vi "Read Name.vi"(8 "error in (no error)":errorcluster, 11 "EmbeddedSMO in":refnum<class "Embedded UI.lvclass">) -> (0 "error out":errorcluster, 2 "Name":string, 3 "EmbeddedSMO out":refnum<class "Embedded UI.lvclass">)   [LabVIEW 2019, in "Embedded UI.lvclass"]
uses:
  Embedded UI.lvclass
  Embedded UI.lvclass/Embedded UI.ctl
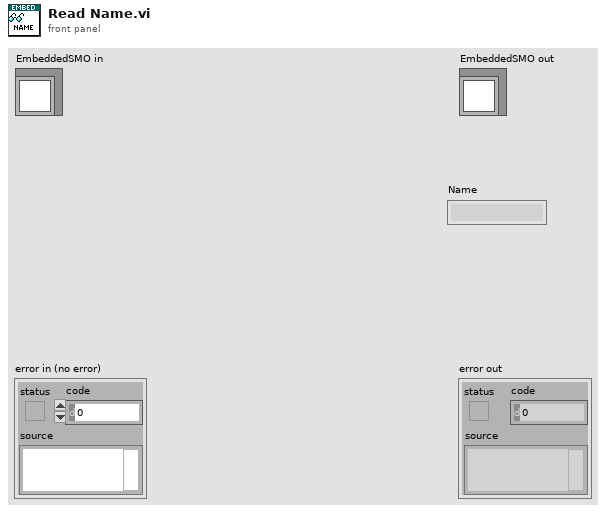
[diagram p1: front panel]
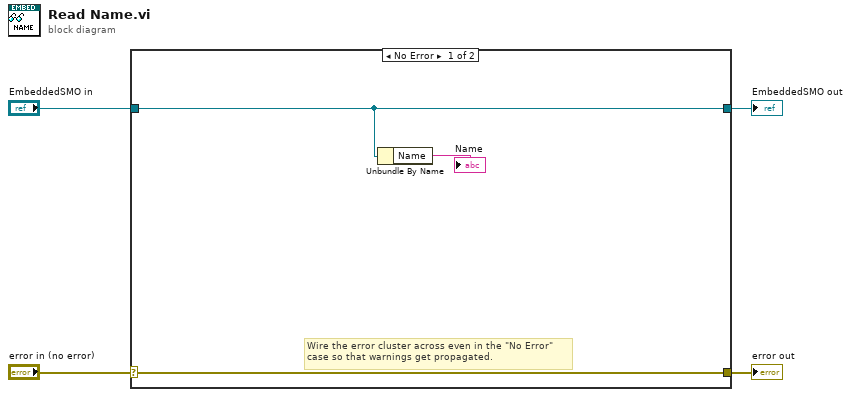
[diagram p0: block diagram]
diagram:
  n1 = case shown="No Error" "error in (no error)" {
    selector: "error in (no error)" -> [w7 w9]
    tunnel: [w7 w9] -> w3
    tunnel: [w6 w8] -> w1
    tunnel: "EmbeddedSMO in" -> [w6 w8]
    frame No Error {
      # "Wire the error cluster across even in the \"No Error\"\ncase so that warnings get propagated."
      n2 = Unbundle By Name(w6) -> ("Name"=→"Name":string)
    }
    frame Error {
    }
  }
  "error out" <- w3
  "EmbeddedSMO out" <- w1
